vi "Handle Type.vi"(7 "Pretty Print?":bool, 8 "error in (no error)":errorcluster, 9 "Type":refnum<class>, 10 "JSON":string, 11 "Flatten To JSON Object in":refnum<class "Generic Object Serializer.lvclass">) -> (0 "error out":errorcluster, 2 "JSON out":string, 3 "Flatten To JSON Object out":refnum<class "Generic Object Serializer.lvclass">)   [LabVIEW 2017, in "Generic Object Serializer.lvclass"]
doc: "Adds type information to the JSON object."
uses:
  Generic Object Serializer/Generic Object Serializer.lvclass
  Generic Object Serializer/Generic Object Serializer.lvclass/Generic Object Serializer.ctl
  Default Serialization Binder/Default Serialization Binder.lvclass
  C:/Users/de200256/Code/logmanoriginal/jsontext-object-serialization/Serialization Binder/Serialization Binder.lvclass
  Serialization Binder/Serialization Binder.lvclass
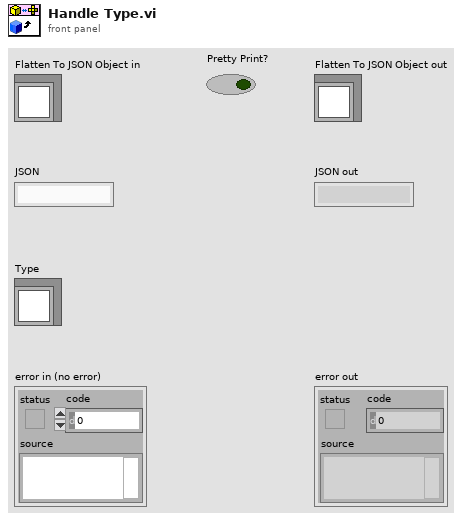
[diagram p1: front panel]
types:
  T1 = typedef "Generic Object Serializer.lvclass/Type Name Handling.ctl" = enum16{"None", "Inline"}
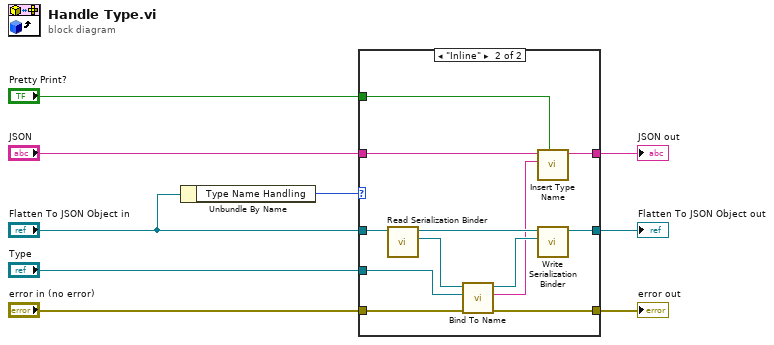
[diagram p0: block diagram]
diagram:
  n1 = Unbundle By Name("Flatten To JSON Object in") -> ("Type Name Handling"=w7:T1)
  n2 = case shown="\"Inline\"" w7 {
    tunnel: [w12 w23] -> w9
    tunnel: "Flatten To JSON Object in" -> [w12 w24]
    tunnel: "Type" -> [_ w22]
    tunnel: "JSON" -> [w11 w16]
    tunnel: [w11 w14] -> w4
    tunnel: "error in (no error)" -> [w10 w18]
    tunnel: [w10 w17] -> w2
    tunnel: "Pretty Print?" -> [_ w13]
    frame Default {
    }
    frame "Inline" {
      n3 = call "Read Serialization Binder.vi"("Flatten To JSON Object in"=w24) -> ("Serialization Binder"=w21:refnum<class "Serialization Binder.lvclass">, "Flatten To JSON Object out"=w19:refnum<class "Generic Object Serializer.lvclass">)  [unwired: 8 in, 1 out]
      n4 = call-dynamic "Bind To Name.vi"("error in (no error)"=w18, "Type"=w22, "Serialization Binder in"=w21) -> ("error out"=w17:errorcluster, "Type Name"=w15:string, "Serialization Binder out"=w20:refnum<class "Serialization Binder.lvclass">)  [unwired: 6 in]
      n5 = call "Insert Type Name.vi"("Pretty Print?"=w13, "Type Name"=w15, "<JSON> in"=w16) -> ("<JSON> out"=w14:string)  [unwired: 8 in]
      n6 = call "Write Serialization Binder.vi"("Serialization Binder"=w20, "Flatten To JSON Object in"=w19) -> ("Flatten To JSON Object out"=w23:refnum<class "Generic Object Serializer.lvclass">)  [unwired: 8 in, 1 out]
    }
  }
  "error out" <- w2
  "Flatten To JSON Object out" <- w9
  "JSON out" <- w4
